vi "ErrCheck_Generic.vi"(8 "Error In":errorcluster, 11 "Macro Command String IN":string="LOOP.Start\t(loop.iterations,3.000);") -> (0 "Error Out":errorcluster, 3 "Undefined GFG Variable? (Warning)":bool)   [LabVIEW 2012]
doc: "SciScan 1.2 160622"
uses:
  <vilib>/Utility/error.llb/whitespace.ctl
  <vilib>/Utility/VariantDataType/Type.ctl
  <vilib>/Utility/VariantDataType/VariantType.lvlib
panel:
  out "Indices of Variables not found":i32[](array[numeric])
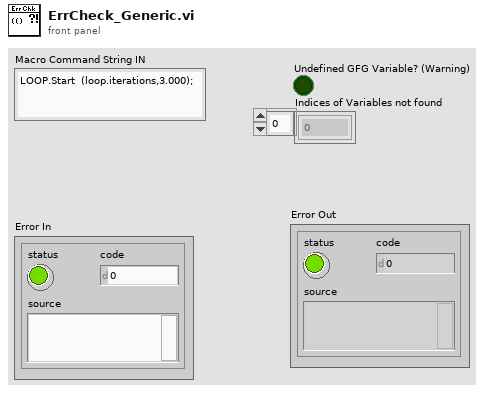
[diagram p1: front panel]
types:
  T1 = typedef "VariantType.lvlib/Type.ctl" = enum8{"Invalid Type", "Void", "I8", "I16", "I32", "I64", "U8", "U16", "U32", "U64", "Single Float", "Double Float", "Extended Float", "Single Complex", "Double Complex", "Extended Complex", "Enum U8", "Enum U16", "Enum U32", "Enum U64", "Single Float With Unit", "Double Float With Unit", "Extended Float With Unit", "Single Complex with Unit", "Double Complex with Unit", "Extended Complex with Unit", "Boolean", "String", "Path", "Picture", "Tag", "Array", "Cluster", "Variant", "LV Variant", "Waveform", "Timestamp", "Digital Waveform", "Digital Data", "ExpressData", "Refnum", "External Data", "VI", "Poly VI", "LabVIEW Class Instance", "Fixed Point"}
  T2 = typedef "whitespace.ctl" = u16
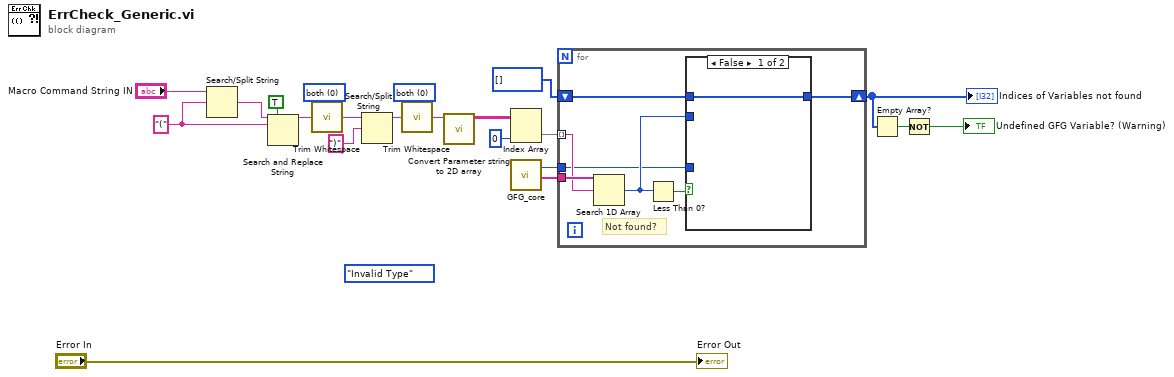
[diagram p0: block diagram]
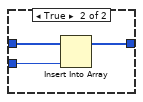
[diagram p2: hidden frame]
diagram:
  (unwired) Type."Invalid Type" ("Data Type Out")
  w13 = T2 0 items=["both", "start of string", "end of string"] ("location (both)")
  w16 = T2 0 items=["both", "start of string", "end of string"] ("location (both)")
  w17 = "(" ("search string/char (-)")
  n1 = Search/Split String(string="Macro Command String IN", search string/char (-)=w17) -> (match + rest of string=w20:string)  [unwired: 1 in, 2 out]
  n2 = Search and Replace String(replace all?=TRUE ("replace all? (F)"), input string=w20, search string=w17) -> (result string=w15:string)  [unwired: 5 in, 3 out]
  n3 = call <vilib>:"Trim Whitespace.vi"("string"=w15, "location (both)"=w16) -> ("trimmed string"=w14:string)
  n4 = Search/Split String(string=w14, search string/char (-)=")") -> (substring before match=w12:string)  [unwired: 1 in, 2 out]
  n5 = call <vilib>:"Trim Whitespace.vi"("string"=w12, "location (both)"=w13) -> ("trimmed string"=w11:string)
  n6 = call "Convert Parameter string to 2D array.vi"("Parameter string IN (without paranthesis)"=w11) -> ("Params table OUT"=w9:string[][])  [unwired: 7 in, 3 out]
  n7 = Index Array(array=w9, index (col)=0 ("disabled index (col)")) -> (element=w7:string[])  [unwired: 1 in]
  n8 = call "GFG_core.vi"() -> ("Data Type Out"=w1:T1, "All Variable Names Out"=w6:string[])  [unwired: 13 in, 5 out]
  n9 = for {
    tunnel: w7 -> [w27] mode=indexing
    tunnel: w6 -> [w28]
    shift-right: [w23] -> w4
    shift-left: i32[] [] -> [w25]
    tunnel: w1 -> [w22]
    # "Not found?"
    n10 = Search 1D Array(1D array=w28, element=w27) -> (index of element=w24:i32)  [unwired: 1 in]
    n11 = Less Than 0?(x=w24) -> (x < 0?=w26:bool)
    n12 = case shown="False" w26 {
      tunnel: w25 -> [w29 w32]
      tunnel: w24 -> [_ w31]
      tunnel: [w29 w30] -> w23
      tunnel: w22 -> [_ _]
      frame False {
      }
      frame True {
        n13 = Insert Into Array(array=w32, new element=w31) -> (w30:i32[])  [unwired: 1 in]
      }
    }
  }
  "Indices of Variables not found" <- w4
  n14 = Empty Array?(array=w4) -> (empty?=w3:bool)
  n15 = Not(x=w3) -> (.not. x?=→"Undefined GFG Variable? (Warning)":bool)
  "Error Out" <- "Error In"
